vi "InitGripper.vi"   [LabVIEW 2020]
doc: "This VI initializes devices related directly to the gripper subsystem."
uses:
  <vilib>/Rock Robotics/SystemInterfaces/i2clib/i2c_bus.ctl
  <vilib>/Rock Robotics/WPI/ThirdParty/REV Robotics/REVLib/Typedef/Color Sensor V3 Resolution.ctl
  <vilib>/Rock Robotics/WPI/ThirdParty/REV Robotics/REVLib/Typedef/Color Sensor V3 MeasurementRate.ctl
  <vilib>/Rock Robotics/WPI/ThirdParty/REV Robotics/REVLib/Typedef/Color Sensor V3 GainFactor.ctl
  <vilib>/Rock Robotics/WPI/Solenoid/WPI_SolenoidChannel.ctl
  GlobalGripper.vi
  <vilib>/Rock Robotics/WPI/Solenoid/WPI_SolenoidOpenDouble.vi
types:
  T1 = typedef "WPI_SolenoidChannel.ctl" = enum8{"Solenoid 0", "Solenoid 1", "Solenoid 2", "Solenoid 3", "Solenoid 4", "Solenoid 5", "Solenoid 6", "Solenoid 7", "Solenoid 8", "Solenoid 9", "Solenoid 10", "Solenoid 11", "Solenoid 12", "Solenoid 13", "Solenoid 14", "Solenoid 15", "Invalid"}
  T2 = typedef "Color Sensor V3 GainFactor.ctl" = enum16{"1x", "3x", "6x", "9x", "18x"}
  T3 = typedef "Color Sensor V3 MeasurementRate.ctl" = enum16{"25ms", "50ms", "100ms", "200ms", "500ms", "1000ms", "2000ms"}
  T4 = typedef "Color Sensor V3 Resolution.ctl" = enum16{"20bit", "19bit", "18bit", "17bit", "16bit", "13bit"}
  T5 = typedef "i2c_bus.ctl" = enum16{"I2C On-Board", "I2C MXP", "Invalid"}
  T6 = typedef "Color Sensor V3 DevRef.ctl" = cluster{"I2CDevRef":T7}
  T7 = typedef "WPI_I2CDevRef.ctl" = cluster{"DevStatus":errorcluster, "Device Address":u8, "Handle":i32, "I2C Bus":T5}
  T8 = typedef "WPI_SolenoidDevRef.ctl" = cluster{"DevStatus":errorcluster, "Pneumatics Control Module":u8, "Forward Solenoid Channel":T1, "Reverse Solenoid Channel":T1}
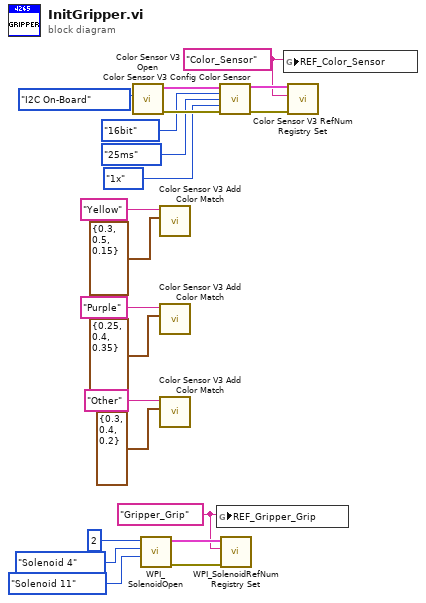
[diagram p0: block diagram]
diagram:
  w4 = "Gripper_Grip" ("refnum name")
  w7 = "Color_Sensor" ("refnum name")
  n1 = call <vilib>:"Color Sensor V3 Open.vi"("I2C Bus"=i2c_bus."I2C On-Board") -> ("error out"=w18:errorcluster, "ColorSensorDevRef"=w20:T6)  [unwired: 9 in]
  n2 = call-poly <vilib>:"WPI_SolenoidOpen.vi"("Reverse Solenoid Channel"=WPI_SolenoidChannel."Solenoid 11", "Forward Solenoid Channel"=WPI_SolenoidChannel."Solenoid 4", "Pneumatics Device (def)"=u8 2) -> ("error out"=w5:errorcluster, "SolenoidDevRef"=w6:T8)  [unwired: 7 in]
  n3 = call <vilib>:"Color Sensor V3 Add Color Match.vi"("Color"=cluster{"R":dbl, "G":dbl, "B":dbl} {"R"=0.3, "G"=0.5, "B"=0.15}, "Name"="Yellow") -> ()  [unwired: 10 in]
  n4 = call <vilib>:"Color Sensor V3 Add Color Match.vi"("Color"=cluster{"R":dbl, "G":dbl, "B":dbl} {"R"=0.25, "G"=0.4, "B"=0.35}, "Name"="Purple") -> ()  [unwired: 10 in]
  n5 = call <vilib>:"Color Sensor V3 Add Color Match.vi"("Color"=cluster{"R":dbl, "G":dbl, "B":dbl} {"R"=0.3, "G"=0.4, "B"=0.2}, "Name"="Other") -> ()  [unwired: 10 in]
  n6 = global write "GlobalGripper.vi" "REF_Gripper_Grip"(w4) -> ()
  n7 = call <vilib>:"Color Sensor V3 Config Color Sensor.vi"("ColorSensorDevRef"=w20, "ColorSensorResolution"=Color_Sensor_V3_Resolution."16bit", "ColorSensorMeasurementRate"=Color_Sensor_V3_MeasurementRate."25ms", "GainFactor"=Color_Sensor_V3_GainFactor."1x", "error in (no error)"=w18) -> ("ColorSensorDevRef out"=w19:T6, "error out"=w17:errorcluster)  [unwired: 9 in]
  n8 = call <vilib>:"WPI_SolenoidRefNum Registry Set.vi"("error in (no error)"=w5, "refnum name"=w4, "SolenoidDevRef"=w6) -> ()  [unwired: 7 in, 2 out]
  n9 = global write "GlobalGripper.vi" "REF_Color_Sensor"(w7) -> ()
  n10 = call <vilib>:"Color Sensor V3 RefNum Registry Set.vi"("error in (no error)"=w17, "refnum name"=w7, "ColorSensorDevRef"=w19) -> ()  [unwired: 7 in, 2 out]
